vi "GET_receive_ServoStatus_fromServo.vi"() -> ()   [LabVIEW 2024]
uses:
  <vilib>/httpClient/ClientHandle.ctl
  DataTypes/OperationTypeForFunctionalGlobalVariable.ctl
  DataTypes/ServoStatus.ctl
  <vilib>/httpClient/LabVIEWHTTPClient.lvlib
panel:
  out "receivedExtractedStatusFromServo":cluster{"mode":string, "position":dbl}
  out "receivedHeadersFromServo":string
  out "receivedBodyFromServo":string
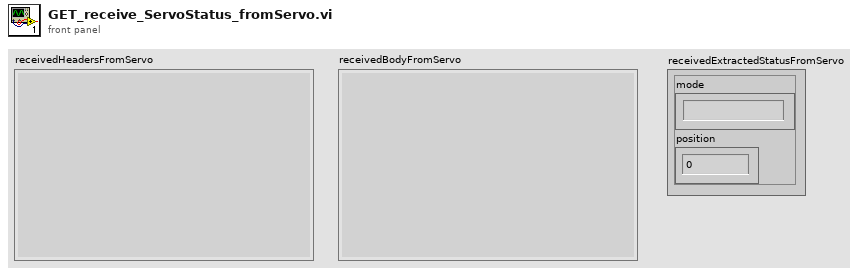
[diagram p1: front panel]
types:
  T1 = typedef "OperationTypeForFunctionalGlobalVariable.ctl" = enum16{"GET", "SET"}
  T2 = typedef "LabVIEWHTTPClient.lvlib/ClientHandle.ctl" = refnum<k1>
  T3 = typedef "ServoStatus.ctl" = cluster{"mode":string, "position":i16}
  T4 = typedef "WebServiceStatus.ctl" = cluster{"isWebServiceShuttingDown":bool}
  T5 = typedef "ServoConnectionParameters.ctl" = cluster{"host":string, "port":u16, "use_https":bool, "timeout_ms":u32, "base_url":string}
  T6 = typedef "ServoConnectionStatus.ctl" = cluster{"esp32Connected":bool}
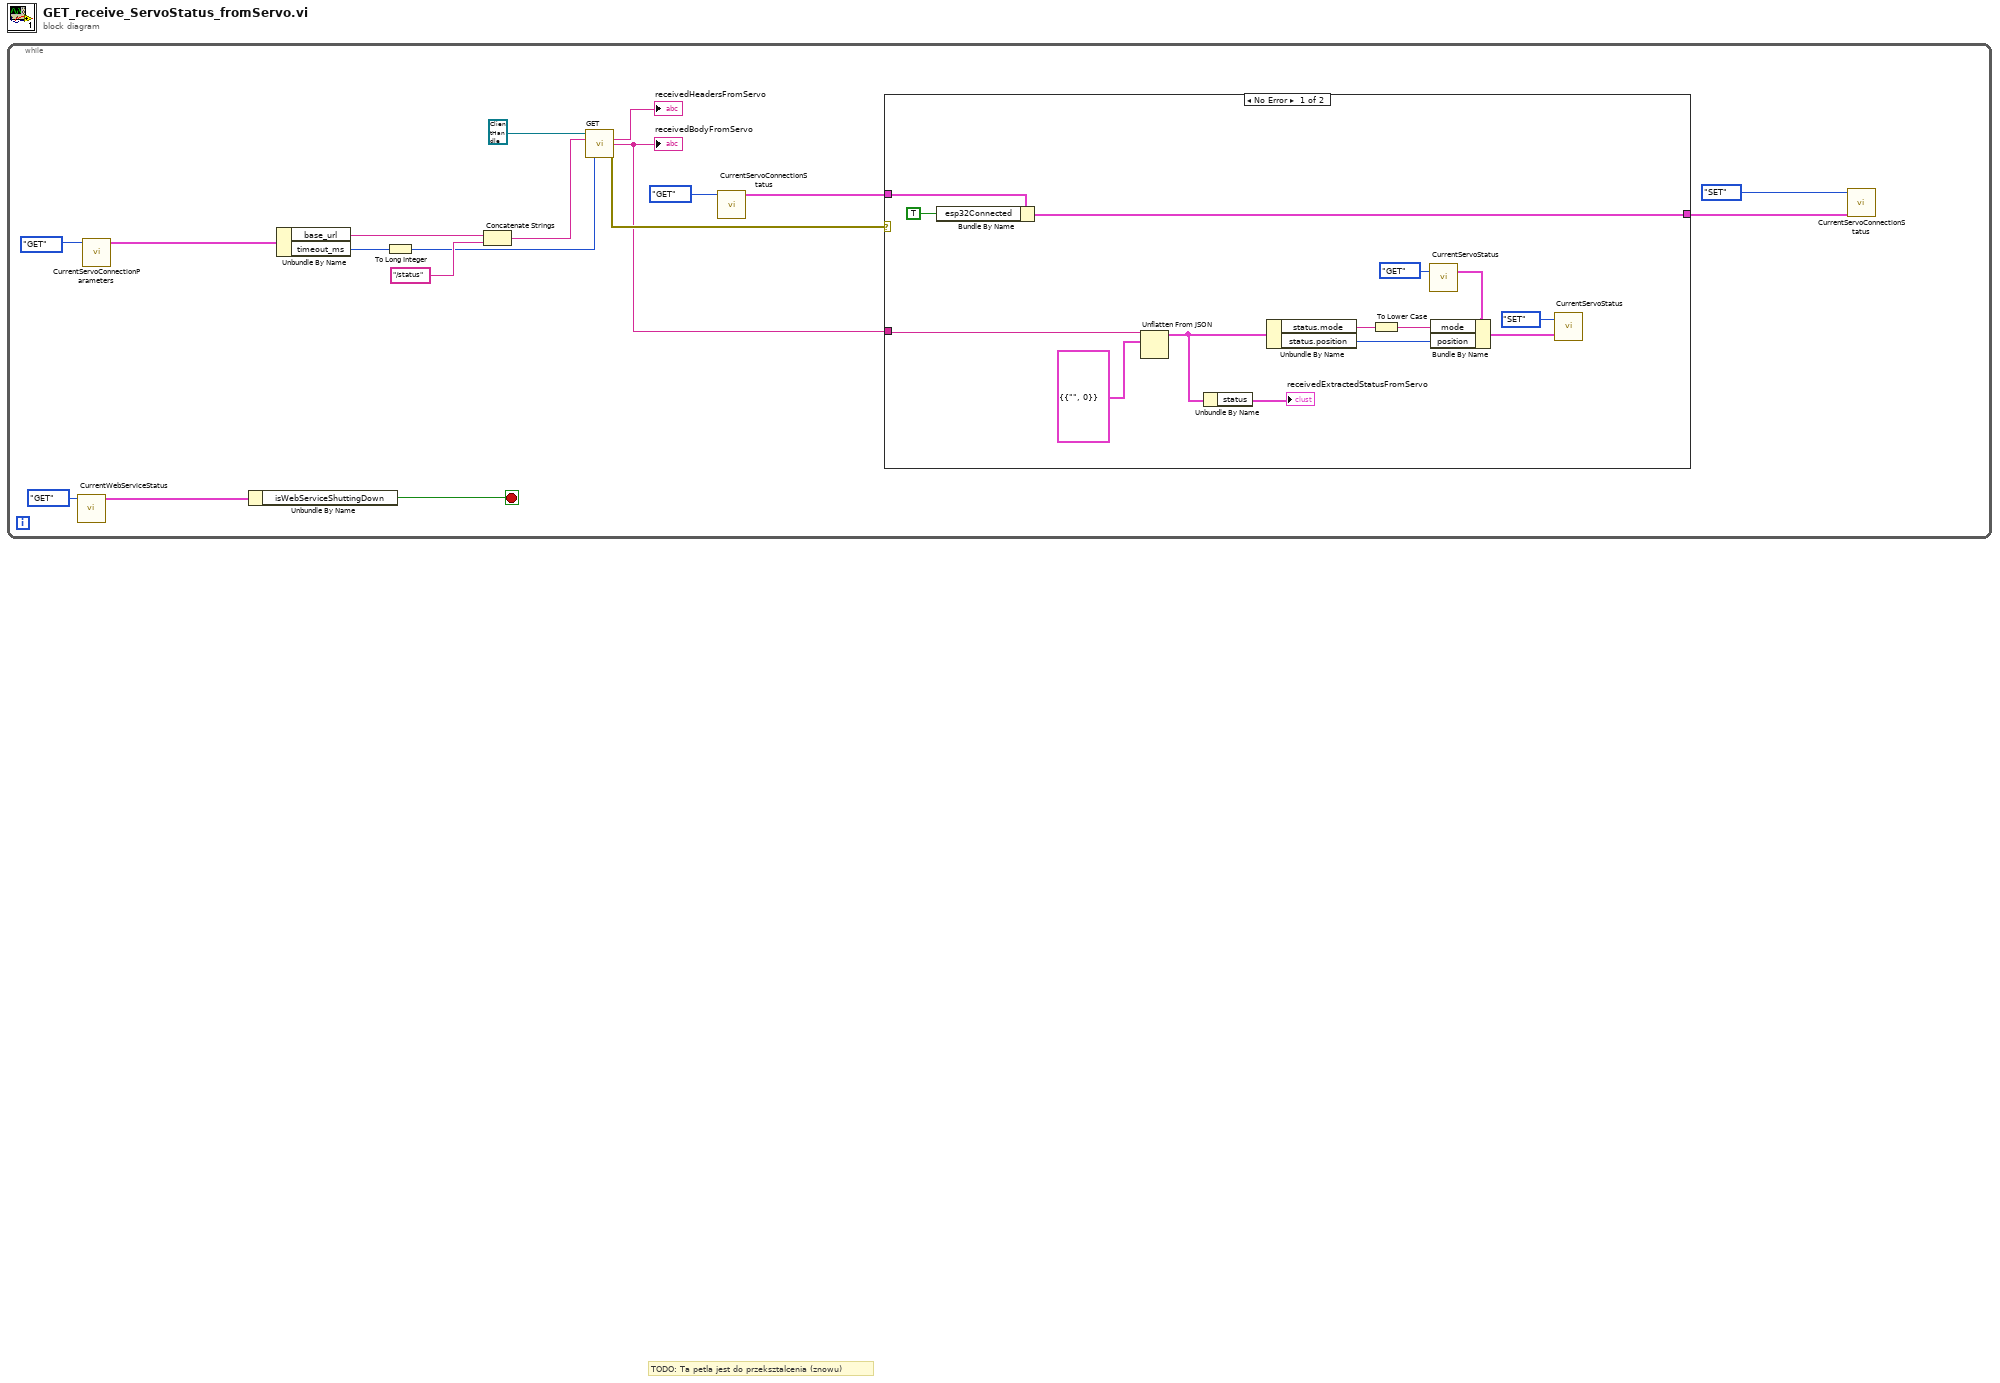
[diagram p0: block diagram]
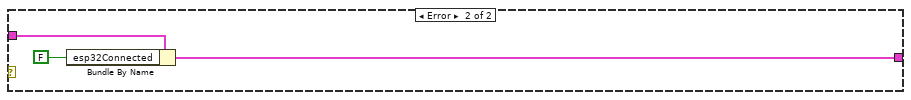
[diagram p2: hidden frame]
diagram:
  # "TODO: Ta petla jest do przeksztalcenia (znowu)"
  n1 = while {
    stop <- w8 stop-if-true
    n2 = call "CurrentWebServiceStatus.vi"("Operation"=OperationTypeForFunctionalGlobalVariable."GET") -> ("Current WebService Status"=w9:T4)  [unwired: 10 in]
    n3 = call "CurrentServoConnectionParameters.vi"("Operation"=OperationTypeForFunctionalGlobalVariable."GET") -> ("Current Servo Connection Parameters"=w17:T5)  [unwired: 10 in]
    n4 = Unbundle By Name(w9) -> ("isWebServiceShuttingDown"=w8:bool)
    n5 = Unbundle By Name(w17) -> ("base_url"=w14:string, "timeout_ms"=w16:u32)
    n6 = To Long Integer(number=w16) -> (32bit integer=w2:i32)
    n7 = Concatenate Strings(w14, "/status" ("string")) -> (w13:string)
    n8 = call <vilib>:"GET.vi"("client handle"=T2 refnum, "url"=w13, "timeout (10000)"=w2) -> ("headers"=→"receivedHeadersFromServo":string, "body"=w1:string, "error out"=w7:errorcluster)  [unwired: 9 in, 1 out]
    "receivedBodyFromServo" <- w1
    n9 = call "CurrentServoConnectionStatus.vi"("Operation"=OperationTypeForFunctionalGlobalVariable."GET") -> ("Current Servo Connection Status"=w6:T6)  [unwired: 10 in]
    n10 = case shown="No Error" w7 {
      tunnel: w6 -> [w31 w34]
      tunnel: [w30 w33] -> w4
      tunnel: w1 -> [w20 _]
      frame No Error {
        n11 = Bundle By Name(cluster=w31, "esp32Connected"=TRUE) -> (w30:T6)
        n12 = Unflatten From JSON(JSON string=w20, type and defaults=cluster{"status":T3} {"status"={"mode"="", "position"=0}}) -> (value=w23:cluster{"status":T3})  [unwired: 5 in, 1 out]
        n13 = Unbundle By Name(w23) -> ("status"=→"receivedExtractedStatusFromServo":T3)
        n14 = Unbundle By Name "Unbundle By Name"(w23) -> ("status.mode"=w28:string, "status.position"=w29:i16)
        n15 = To Lower Case(string=w28) -> (all lower case string=w27:string)
        n16 = call "CurrentServoStatus.vi"("Operation"=OperationTypeForFunctionalGlobalVariable."GET") -> ("Current Servo Status"=w21:T3)  [unwired: 2 in]
        n17 = Bundle By Name(cluster=w21, "mode"=w27, "position"=w29) -> (w24:T3)
        n18 = call "CurrentServoStatus.vi"("New Servo Status"=w24, "Operation"=OperationTypeForFunctionalGlobalVariable."SET") -> ()  [unwired: 1 in, 1 out]
      }
      frame Error {
        n19 = Bundle By Name(cluster=w34, "esp32Connected"=FALSE) -> (w33:T6)
      }
    }
    n20 = call "CurrentServoConnectionStatus.vi"("New Servo Connection Status"=w4, "Operation"=OperationTypeForFunctionalGlobalVariable."SET") -> ()  [unwired: 9 in, 1 out]
  }
